vi "main.vi"() -> ()   [LabVIEW 2023]
uses:
  CONTROLS/Control 1.ctl
panel:
  out "Meldung":string
  out "Enum":T1
  in  "stop":bool
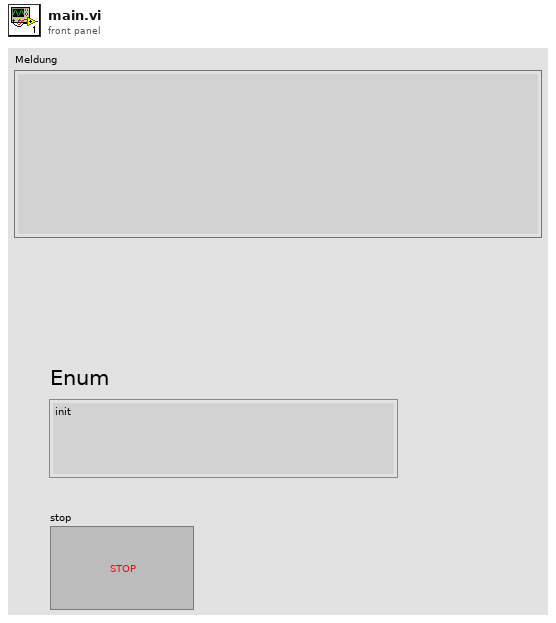
[diagram p1: front panel]
types:
  T1 = typedef "Control 1.ctl" = enum16{"init", "read", "write", "Kundeneingabe", "Betonauswahl", "Bezahlprozess", "Rechnung", "Zudaten mit Gewichtmessung", "Stop"}
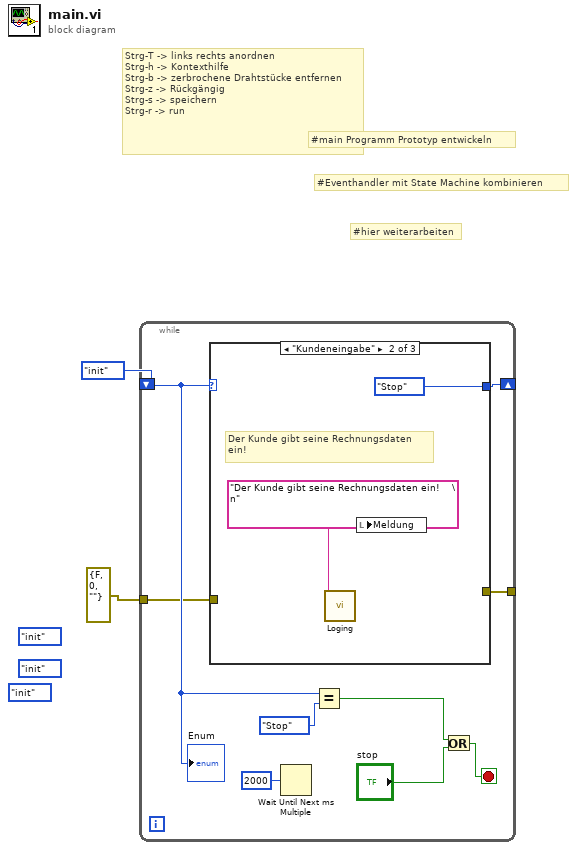
[diagram p0: block diagram]
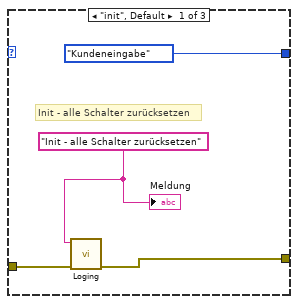
[diagram p2: hidden frame]
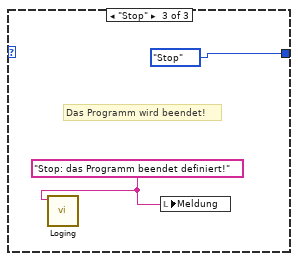
[diagram p3: hidden frame]
diagram:
  (unwired) Control_1."init"
  (unwired) Control_1."init"
  (unwired) Control_1."init"
  # "#hier weiterarbeiten"
  # "#Eventhandler mit State Machine kombinieren"
  # "#main Programm Prototyp entwickeln"
  # "Strg-T -> links rechts anordnen\nStrg-h -> Kontexthilfe\nStrg-b -> zerbrochene Drahtstücke entfernen\nStrg-z -> Rückgängig\nStrg-s -> speichern\nStrg-r -> run"
  n1 = while {
    shift-right: [w11] -> _
    shift-left: Control_1."init" -> [w9]
    tunnel: [w4] -> _
    tunnel: errorcluster {"status"=FALSE, "code"=0, "source"=""} ("error in") -> [w3]
    stop <- w6 stop-if-true
    n2 = case shown="\"Kundeneingabe\"" w9 {
      tunnel: [Control_1."Kundeneingabe" Control_1."Stop" Control_1."Stop"] -> w11
      tunnel: [w13 _ _] -> w4
      tunnel: w3 -> [w12 _ _]
      frame "init", Default {
        w14 = "Init - alle Schalter zurücksetzen" ("Meldung")
        # "Init - alle Schalter zurücksetzen"
        n3 = call "Loging.vi"("error in"=w12, "log"=w14) -> ("error out"=w13:errorcluster)  [unwired: 9 in]
        "Meldung" <- w14
      }
      frame "Kundeneingabe" {
        w16 = "Der Kunde gibt seine Rechnungsdaten ein!    \n" ("Meldung")
        # "Der Kunde gibt seine Rechnungsdaten \nein!"
        n4 = call "Loging.vi"("log"=w16) -> ()  [unwired: 10 in, 1 out]
        n5 = local write "Meldung"(w16) -> ()
      }
      frame "Stop" {
        w18 = "Stop: das Programm beendet definiert!" ("Meldung")
        # "Das Programm wird beendet!"
        n6 = call "Loging.vi"("log"=w18) -> ()  [unwired: 10 in, 1 out]
        n7 = local write "Meldung"(w18) -> ()
      }
    }
    n8 = Wait Until Next ms Multiple(millisecond multiple=u32 2000) -> ()  [unwired: 1 out]
    n9 = Equal?(x=w9, y=Control_1."Stop") -> (x = y?=w8:bool)
    n10 = Or(x=w8, y="stop") -> (x .or. y?=w6:bool)
    "Enum" <- w9
  }
